vi "Create queues.vi"(8 "error in (no error)":errorcluster, 10 "timeout":i32, 11 "Messenger in":refnum<class "Messenger.lvclass">) -> (0 "error out":errorcluster, 3 "Messenger out":refnum<class "Messenger.lvclass">)   [LabVIEW 2018, in "Messenger.lvclass"]
uses:
  Messenger.lvclass
  Custom/S4msg.ctl
  Messenger.lvclass/Messenger.ctl
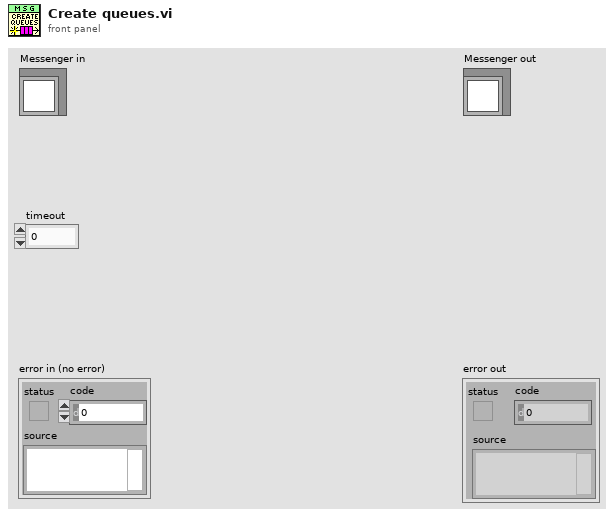
[diagram p1: front panel]
types:
  T1 = typedef "S4msg.ctl" = cluster{"msg topic":string, "msg data":variant}
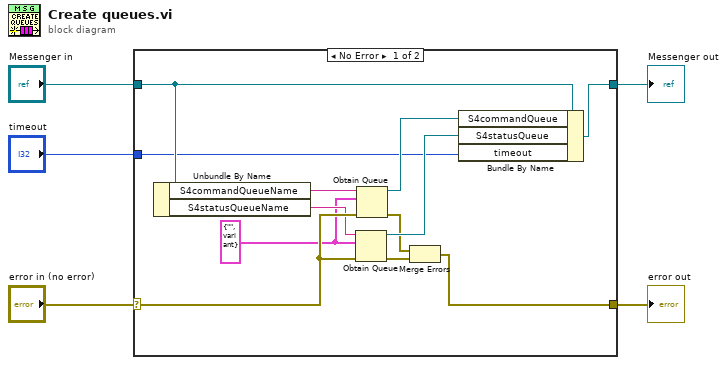
[diagram p0: block diagram]
diagram:
  n1 = case shown="No Error" "error in (no error)" {
    selector: "error in (no error)" -> [w17 w18]
    tunnel: [w9 w18] -> w4
    tunnel: [w8 w19] -> w2
    tunnel: "Messenger in" -> [w14 w19]
    tunnel: "timeout" -> [w7 _]
    frame No Error {
      w6 = T1 {"msg topic"="", "msg data"=variant} ("S4msg")
      n2 = Unbundle By Name(w14) -> ("S4commandQueueName"=w15:string, "S4statusQueueName"=w16:string)
      n3 = Obtain Queue(name (unnamed)=w16, element data type=w6, error in (no error)=w17) -> (queue out=w12:refnum<queue>, error out=w11:errorcluster)  [unwired: 2 in, 1 out]
      n4 = Obtain Queue(name (unnamed)=w15, element data type=w6, error in (no error)=w17) -> (queue out=w13:refnum<queue>, error out=w10:errorcluster)  [unwired: 2 in, 1 out]
      n5 = Merge Errors(w10, w11) -> (w9:errorcluster)
      n6 = Bundle By Name(cluster=w14, "S4commandQueue"=w13, "S4statusQueue"=w12, "timeout"=w7) -> (w8:refnum<class "Messenger.lvclass">)
    }
    frame Error {
    }
  }
  "error out" <- w4
  "Messenger out" <- w2
